vi "flipud.vi"(10 "dimension":i32=1, 11 "Array":u16[][](array[numeric])) -> (3 "Fliped Up Down":u16[][](array[numeric]))   [LabVIEW 2015]
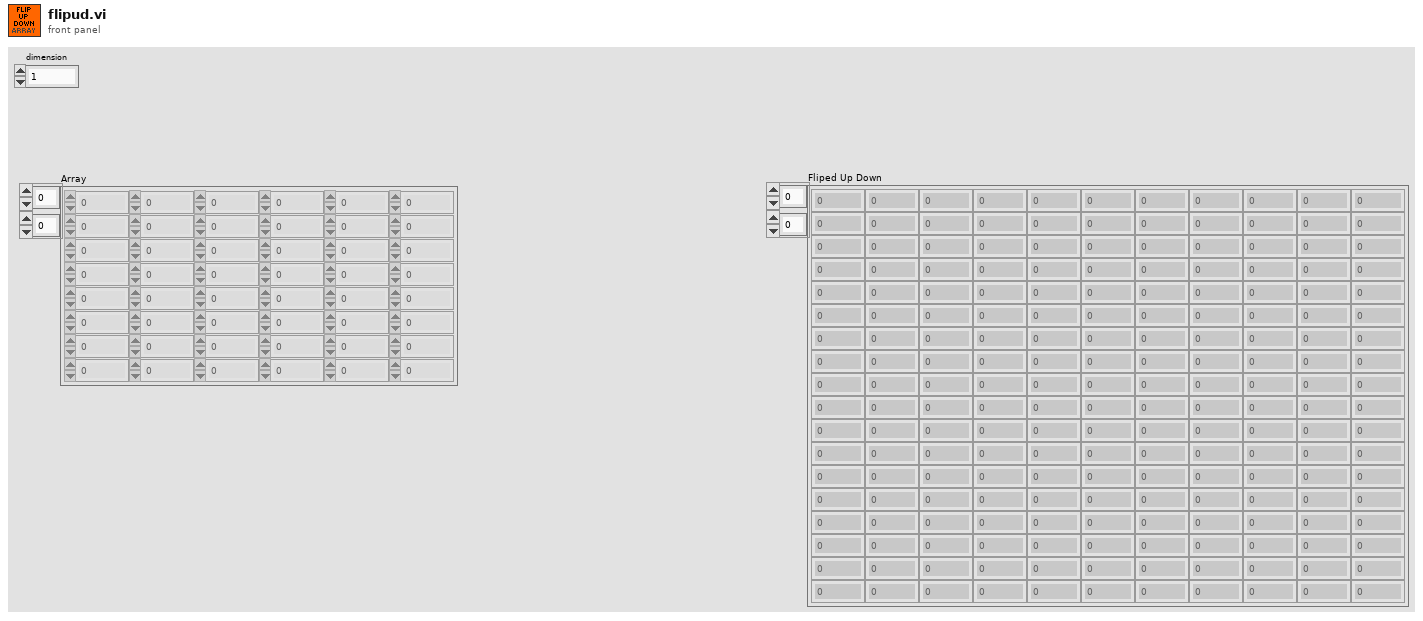
[diagram p1: front panel]
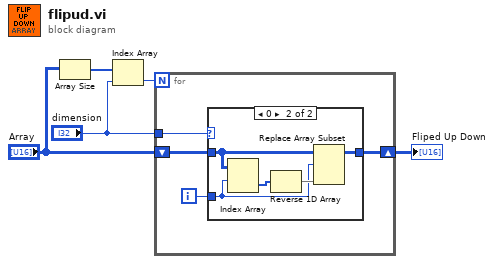
[diagram p0: block diagram]
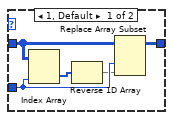
[diagram p2: hidden frame]
diagram:
  n1 = Array Size(array="Array") -> (size(s)=w5:i32[])
  n2 = Index Array(array=w5, index="dimension") -> (element=w4:i32)
  n3 = for {
    N: w4 -> [_]
    shift-right: [w7] -> w3
    shift-left: "Array" -> [w9]
    tunnel: "dimension" -> [w6]
    i -> [w8]
    n4 = case shown="0" w6 {
      tunnel: w9 -> [w13 w18]
      tunnel: w8 -> [w12 w15]
      tunnel: [w10 w16] -> w7
      frame 1, Default {
        n5 = Index Array(array=w13, index (col)=w12) -> (element=w14:u16[])  [unwired: 1 in]
        n6 = Reverse 1D Array(array=w14) -> (reversed array=w11:u16[])
        n7 = Replace Array Subset(array=w13, new element=w11, index (col)=w12) -> (w10:u16[][])  [unwired: 1 in]
      }
      frame 0 {
        n8 = Index Array(array=w18, index (row)=w15) -> (element=w19:u16[])  [unwired: 1 in]
        n9 = Reverse 1D Array(array=w19) -> (reversed array=w17:u16[])
        n10 = Replace Array Subset(array=w18, new element=w17, index (row)=w15) -> (w16:u16[][])  [unwired: 1 in]
      }
    }
  }
  "Fliped Up Down" <- w3
